vi "Add Ticks to PUC.vi"(1 "Ticks Calibrated s's":ext[](array[numeric]), 2 "Ticks Calibrated g's":ext[](array[numeric]), 3 "Ticks Lifetimes":ext[](array[numeric]), 5 "Lifetime Array in":ext[](array[numeric]), 7 "Calibrated g Array in":ext[](array[numeric]), 9 "Calibrated s Array in":ext[](array[numeric]), 11 "error in (no error)":errorcluster, 12 "Tick Length":dbl=0.01) -> (6 "Lifetime Array out":ext[](array[numeric]), 8 "Calibrated g Array out":ext[](array[numeric]), 10 "Calibrated s Array out":ext[](array[numeric]), 15 "error out":errorcluster)   [LabVIEW 2019]
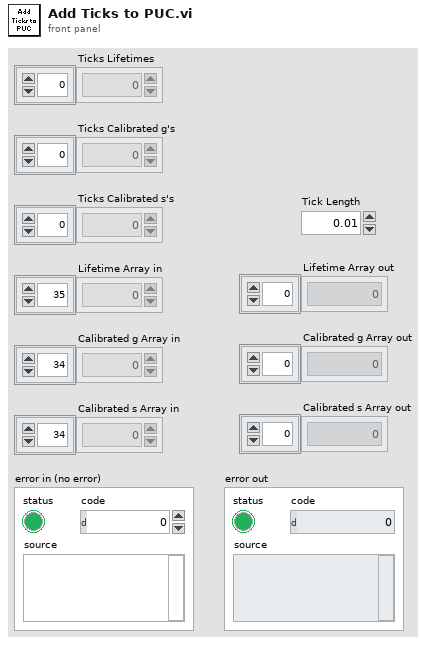
[diagram p1: front panel]
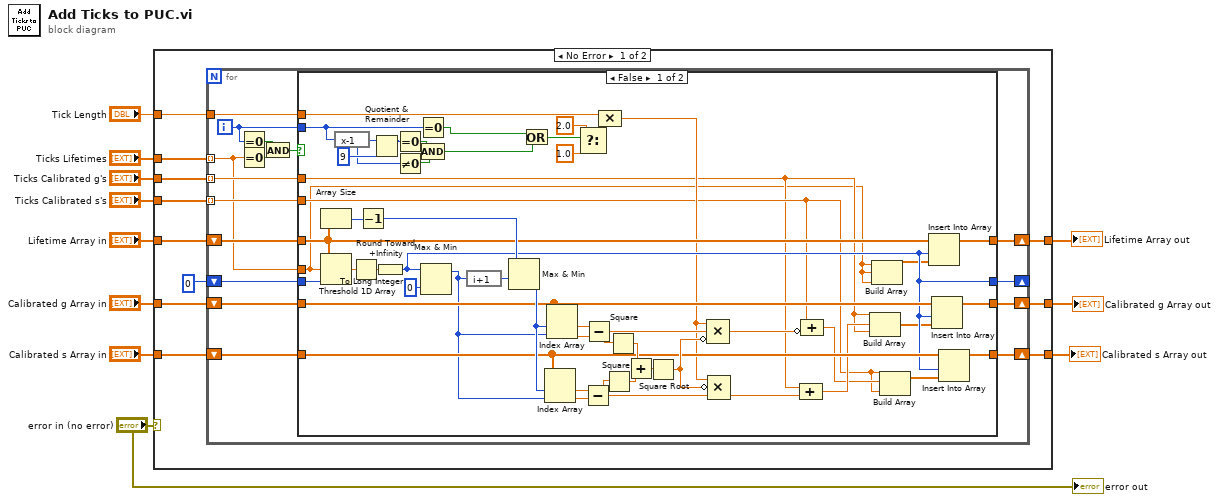
[diagram p0: block diagram]
diagram:
  n1 = case shown="No Error" "error in (no error)" {
    tunnel: "Ticks Lifetimes" -> [w22 _]
    tunnel: "Ticks Calibrated g's" -> [w21 _]
    tunnel: "Ticks Calibrated s's" -> [w20 _]
    tunnel: "Lifetime Array in" -> [w19 w95]
    tunnel: "Calibrated g Array in" -> [w18 w94]
    tunnel: "Calibrated s Array in" -> [w17 w93]
    tunnel: [w16 w95] -> w5
    tunnel: [w15 w94] -> w4
    tunnel: [w14 w93] -> w3
    tunnel: "Tick Length" -> [w12 _]
    frame No Error {
      n2 = for {
        tunnel: w22 -> [w27] mode=indexing
        tunnel: w21 -> [w28] mode=indexing
        tunnel: w20 -> [w29] mode=indexing
        shift-right: [w33] -> w16
        shift-left: w19 -> [w34]
        shift-right: [w35] -> w15
        shift-left: w18 -> [w36]
        shift-right: [w31] -> w14
        shift-left: w17 -> [w32]
        shift-right: [w30] -> _
        shift-left: 0 -> [w38]
        tunnel: w12 -> [w37]
        i -> [w26]
        n3 = Equal To 0?(x=w26) -> (x = 0?=w25:bool)
        n4 = Equal To 0?(x=w27) -> (x = 0?=w24:bool)
        n5 = And(x=w25, y=w24) -> (x .and. y?=w23:bool)
        n6 = case shown="False" w23 {
          tunnel: w38 -> [w88 w91]
          tunnel: w37 -> [w68 _]
          tunnel: w36 -> [w60 w90]
          tunnel: [w59 w90] -> w35
          tunnel: w34 -> [w58 w92]
          tunnel: [w57 w92] -> w33
          tunnel: w32 -> [w56 w89]
          tunnel: [w55 w89] -> w31
          tunnel: [w54 w91] -> w30
          tunnel: w27 -> [w41 _]
          tunnel: w29 -> [w46 _]
          tunnel: w28 -> [w45 _]
          tunnel: w26 -> [w69 _]
          frame False {
            n7 = Array Size(array=w58) -> (size(s)=w86:i32)
            n8 = Threshold 1D Array(1:w88, 2:w41, 3:w58) -> (0:w40:ext)
            n9 = expression code="x-1"(w69) -> (w76:i32)
            n10 = Round Toward +Infinity(x=w40) -> (ceil(x): smallest int >= x=w39:ext)
            n11 = Decrement(x=w86) -> (x-1=w85:i32)
            n12 = Quotient & Remainder(x=w76, y=9 ("# Decades")) -> (x-y*floor(x/y)=w71:i32)  [unwired: 1 out]
            n13 = To Long Integer(number=w39) -> (32bit integer=w54:i32)
            n14 = Equal To 0?(x=w71) -> (x = 0?=w75:bool)
            n15 = Not Equal To 0?(x=w76) -> (x != 0?=w78:bool)
            n16 = Equal To 0?(x=w69) -> (x = 0?=w43:bool)
            n17 = Max & Min(x=w54, y=0) -> (max(x,y)=w44:i32)  [unwired: 1 out]
            n18 = Compound Arithmetic op=AND(w75, w78) -> (w77:bool)
            n19 = expression code="i+1"(w44) -> (w42:i32)
            n20 = Max & Min(x=w85, y=w42) -> (min(x,y)=w84:i32)  [unwired: 1 out]
            n21 = Or(x=w43, y=w77) -> (x .or. y?=w70:bool)
            n22 = Index Array(array=w56, index #1=w84, index #2=w44) -> (element #1=w81:ext, element #2=w80:ext)
            n23 = Index Array(array=w60, index #1=w84, index #2=w44) -> (element #1=w83:ext, element #2=w82:ext)
            n24 = Select(t=2.0 ("value"), s=w70, f=1.0) -> (s? t:f=w74:dbl)
            n25 = Subtract(x=w81, y=w80) -> (x-y=w63:ext)
            n26 = Subtract(x=w83, y=w82) -> (x-y=w64:ext)
            n27 = Compound Arithmetic op=MULTIPLY(w68, w74) -> (w53:dbl)
            n28 = Square(x=w63) -> (x^2=w67:ext)
            n29 = Square(x=w64) -> (x^2=w66:ext)
            n30 = Add(x=w66, y=w67) -> (x+y=w65:ext)
            n31 = Square Root(x=w65) -> (sqrt(x)=w62:ext)
            n32 = Compound Arithmetic op=MULTIPLY(w53, w64, invert w62) -> (w52:ext)
            n33 = Compound Arithmetic op=MULTIPLY(w53, invert w62, w63) -> (w61:ext)
            n34 = Compound Arithmetic op=ADD(w45, w61) -> (w48:ext)
            n35 = Compound Arithmetic op=ADD(w46, invert w52) -> (w47:ext)
            n36 = Build Array(w45, w48, w45) -> (w50:ext[])
            n37 = Build Array(w41, w41, w41) -> (w51:ext[])
            n38 = Build Array(w46, w47, w46) -> (w49:ext[])
            n39 = Insert Into Array(array=w58, index=w54, new element=w51) -> (w57:ext[])
            n40 = Insert Into Array(array=w60, index=w54, new element=w50) -> (w59:ext[])
            n41 = Insert Into Array(array=w56, index=w54, new element=w49) -> (w55:ext[])
          }
          frame True {
            # "skip first tick if tau = 0, as it is sometimes problematic"
          }
        }
      }
    }
    frame Error {
    }
  }
  "Calibrated s Array out" <- w3
  "Calibrated g Array out" <- w4
  "Lifetime Array out" <- w5
  "error out" <- "error in (no error)"
